vi "Buffer.Read.1D.U8.vi"(7 "count":i64 format="%d elements", 8 "error in (no error)":errorcluster, 9 "offset (0)":u64 format="%d bytes", 10 "buffer in":u8[](array[numeric]), 11 "Buffer in":refnum<class "Buffer.lvclass">) -> (0 "error out":errorcluster, 1 "offset out":u64 format="%d bytes", 2 "buffer out":u8[](array[numeric]), 3 "Buffer out":refnum<class "Buffer.lvclass">)   [LabVIEW 2017, in "DSF Core.lvlib" / "Buffer.lvclass"]
uses:
  Buffer.lvclass
  C:/Program Files (x86)/National Instruments/LabVIEW 2017/vi.lib/NI/Memory Manager/Classes/Pointer/Memory.Pointer.lvclass
  <vilib>/NI/Memory Manager/Classes/Pointer/Memory.Pointer.lvclass/Memory.Pointer.ctl
  <vilib>/NI/Memory Manager/Classes/Pointer/Memory.Pointer.Read.1D.U8.vi
  <vilib>/NI/Memory Manager/Classes/Pointer/Memory.Pointer.Read.No Check.1D.U8.vi
  <vilib>/NI/Memory Manager/Classes/Pointer/Memory.Pointer.Parameter Check.Null Pointer.vi
  <vilib>/NI/Memory Manager/Classes/Pointer/Memory.Pointer.Parameter Check.Subset.Power of 2.vi
  <vilib>/NI/Memory Manager/Classes/Pointer/Memory.Pointer.Get Address.vi
  <vilib>/NI/Memory Manager/Classes/Pointer/Memory.Pointer.Errors.vi
  <vilib>/NI/Memory Manager/Classes/Pointer/Memory.Pointer.Errors.Null Pointer.vi
  <vilib>/NI/Memory Manager/Classes/Pointer/Memory.Pointer.Errors.Out of Bounds.vi
  <vilib>/NI/Memory Manager/Classes/Pointer/Memory.Pointer.Get Size.vi
  <vilib>/NI/Memory Manager/Classes/Pointer/Memory.Pointer.Count to Size.Power of 2.vi
  <vilib>/NI/Memory Manager/Classes/Pointer/Memory.Pointer.Errors.Create Error.vi
  <vilib>/NI/Memory Manager/VIs/Source.Write.String.vi
  <vilib>/NI/Memory Manager/Classes/Pointer/Memory.Pointer.Errors.Write Pointer Size.vi
  <vilib>/NI/Memory Manager/VIs/Source.Write.Scalar.Base10.vi
  <vilib>/NI/Memory Manager/VIs/Source.Write.Scalar.Base10 (U64).vi
  <vilib>/NI/Memory Manager/VIs/New Error Cluster Constant.vi
  <vilib>/NI/Memory Manager/VIs/New Error Cluster Constant (512B).vi
  <vilib>/NI/Memory Manager/VIs/Error Cluster.Set Status.vi
  <vilib>/NI/Memory Manager/VIs/Error Cluster.Set Code.vi
  <vilib>/NI/Memory Manager/VIs/Error Cluster.Set VI Source.vi
  <vilib>/NI/Memory Manager/Constants/Memory.Constants.vi
  <vilib>/NI/Memory Manager/Constants/Memory.Constants.Library Name.vi
  <vilib>/NI/Memory Manager/Classes/Pointer/Memory.Pointer.Errors.Get Info.vi
  <vilib>/NI/Memory Manager/Classes/Pointer/Memory.Pointer.lvclass
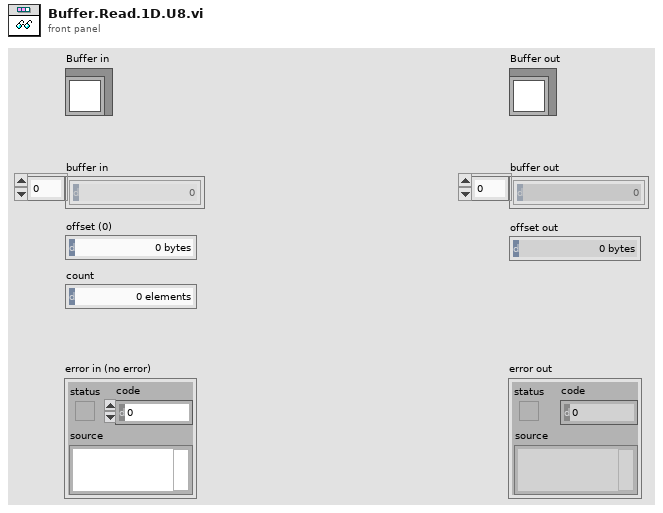
[diagram p1: front panel]
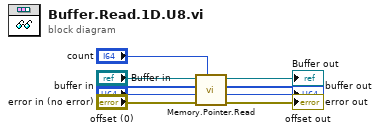
[diagram p0: block diagram]
diagram:
  n1 = call-poly <vilib>:"Memory.Pointer.Read.vi"("count (-1: all)"="count", "error in (no error)"="error in (no error)", "offset (0)"="offset (0)", "buffer in"="buffer in", "Pointer in"="Buffer in") -> ("error out"=→"error out":errorcluster, "offset out"=→"offset out":u64, "buffer out"=→"buffer out":u8[], "Pointer out"=→"Buffer out":refnum<class "Buffer.lvclass">)  [unwired: 3 in]
